vi "Main.vi"(8 "Error In":errorcluster) -> (0 "Error Out":errorcluster)   [LabVIEW 2017, in "Controller.lvlib"]
uses:
  Controller.lvlib
  InternalData.ctl
  UserEvents/StopUE.lvlib
  ErrorHandler/ErrorHandler.lvlib
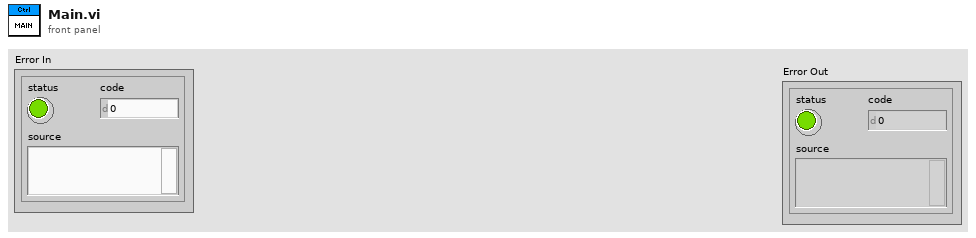
[diagram p1: front panel]
types:
  T1 = typedef "Controller.lvlib/InternalData.ctl" = cluster{"Status":string}
  T2 = typedef "Controller.lvlib/States_Module.ctl" = enum16{"DoSomething", "Shutdown", "Initialize"}
  T3 = typedef "Controller.lvlib/MessageData.ctl" = cluster{"State":T2, "Payload":variant, "WaitOnReply":bool, "ReplyNotif":refnum<notifier>}
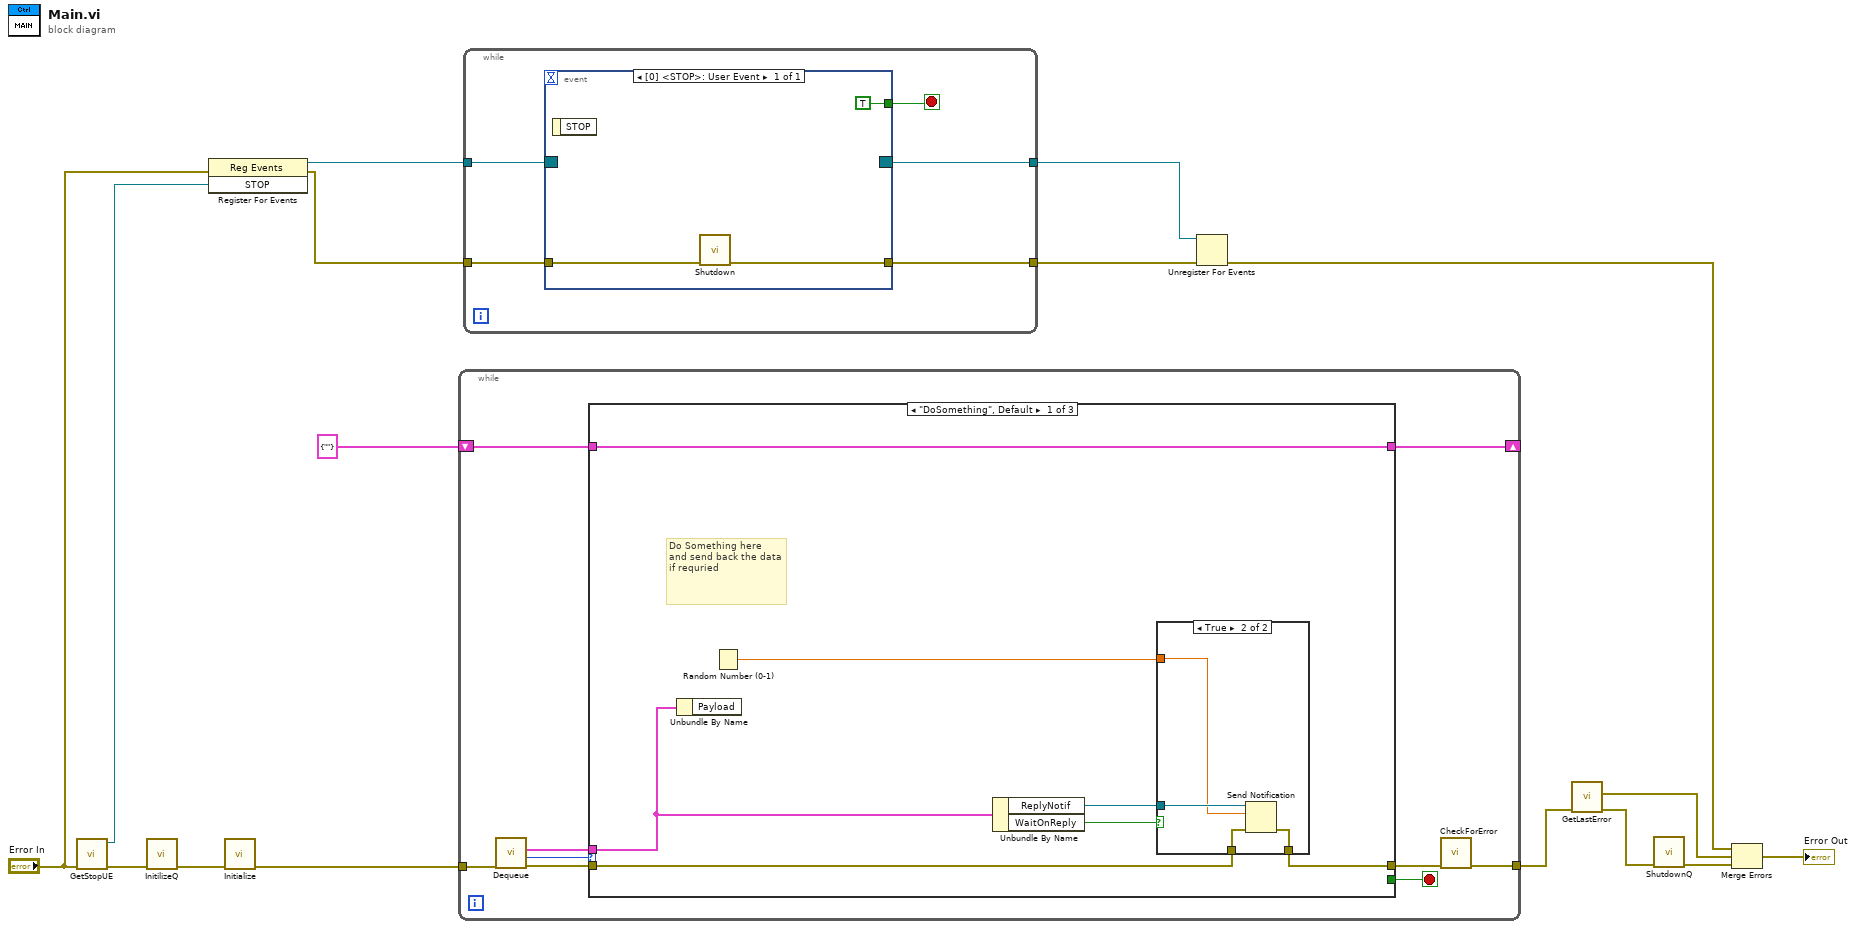
[diagram p0: block diagram]
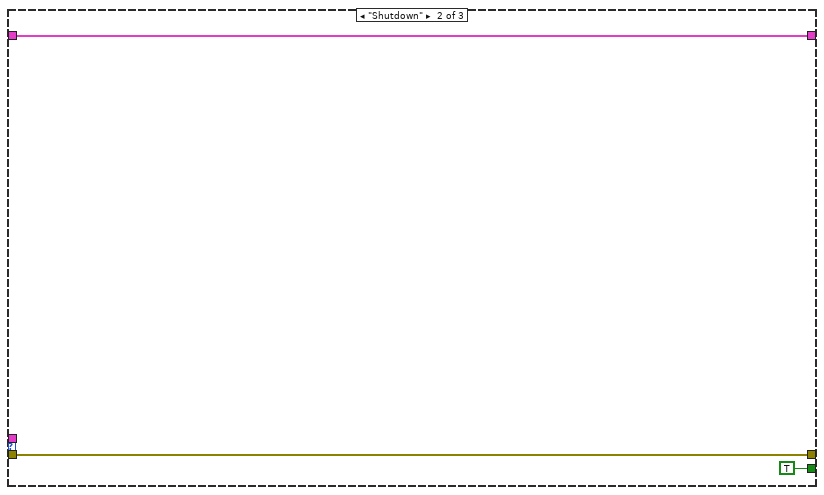
[diagram p3: hidden frame]
diagram:
  n1 = call "GetStopUE.vi"("Error In"="Error In") -> ("Error Out"=w13:errorcluster, "STOP"=w16:refnum<user-event>)  [unwired: 9 in]
  n2 = call "InitilizeQ.vi"("Error In"=w13) -> ("Error Out"=w11:errorcluster)  [unwired: 10 in]
  n3 = register-events(error in="Error In", w16) -> (reference out=w15:refnum<event-registration>, error out=w14:errorcluster)  [unwired: 1 in]
  n4 = call "Initialize.vi"("Error In"=w11) -> ("error out"=w10:errorcluster)  [unwired: 9 in, 1 out]
  n5 = while {
    tunnel: w10 -> [w25]
    tunnel: [w18] -> w7
    shift-right: [w20] -> _
    shift-left: T1 {"Status"=""} ("InternalData") -> [w21]
    stop <- w22 stop-if-true
    n6 = call "Dequeue.vi"("Error In"=w25) -> ("error out"=w24:errorcluster, "State"=w23:T2, "Data out"=w17:T3)  [unwired: 8 in]
    n7 = case shown="\"DoSomething\", Default" w23 {
      tunnel: w24 -> [w31 w39 w42]
      tunnel: [_ TRUE _] -> w22
      tunnel: [w30 w39 w42] -> w19
      tunnel: w21 -> [w32 w38 w41]
      tunnel: [w32 w38 w41] -> w20
      tunnel: w17 -> [w28 _ _]
      frame "DoSomething", Default {
        # "Do Something here\nand send back the data if requried"
        n8 = Unbundle By Name(w28) -> ()  [unwired: 1 out]
        n9 = Random Number (0-1)() -> (number: 0 to 1=w29:dbl)
        n10 = Unbundle By Name(w28) -> ("ReplyNotif"=w26:refnum<notifier>, "WaitOnReply"=w27:bool)
        n11 = case shown="True" w27 {
          tunnel: w31 -> [w33 w37]
          tunnel: [w33 w36] -> w30
          tunnel: w26 -> [_ w35]
          tunnel: w29 -> [_ w34]
          frame False {
          }
          frame True {
            n12 = Send Notification(notification=w34, notifier=w35, error in (no error)=w37) -> (error out=w36:errorcluster)  [unwired: 1 out]
          }
        }
      }
      frame "Shutdown" {
      }
      frame "Initialize" {
      }
    }
    n13 = call "CheckForError.vi"("Error In"=w19) -> ("error out"=w18:errorcluster)  [unwired: 10 in]
  }
  n14 = while {
    tunnel: w15 -> [w47]
    tunnel: w14 -> [w45]
    tunnel: [w44] -> w9
    tunnel: [w43] -> w8
    stop <- w46 stop-if-true
    n15 = event shown="[0] <STOP>: User Event" {
      selector: w47 -> [_]
      dyn-events: [_] -> w43
      timeout: _ -> [_]
      tunnel: [TRUE] -> w46
      tunnel: w45 -> [w49]
      tunnel: [w48] -> w44
      event User Event {
        n16 = event-data() -> ()  [unwired: 1 in, 1 out]
        n17 = call "Shutdown.vi"("Error In"=w49) -> ("error out"=w48:errorcluster)  [unwired: 9 in, 1 out]
      }
    }
  }
  n18 = Unregister For Events(event registration refnum=w8, error in=w9) -> (error out=w3:errorcluster)
  n19 = call "GetLastError.vi"("Error In"=w7) -> ("error IO"=w6:errorcluster, "Last Error"=w4:errorcluster)  [unwired: 9 in]
  n20 = call "ShutdownQ.vi"("Error In"=w6) -> ("Error Out"=w5:errorcluster)  [unwired: 10 in]
  n21 = Merge Errors(w3, w4, w5) -> (→"Error Out":errorcluster)
